vi "LogScaledMessagesOutput.vi"(11 "data out":dbl[](array[numeric])) -> ()   [LabVIEW 2015, in "Diagnostics Addon Engine.lvlib"]
uses:
  Diagnostics Addon Engine.lvlib
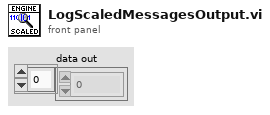
[diagram p1: front panel]
types:
  T1 = enum16{"open", "replace", "create", "open or create", "replace or create", "replace or create with confirmation"}
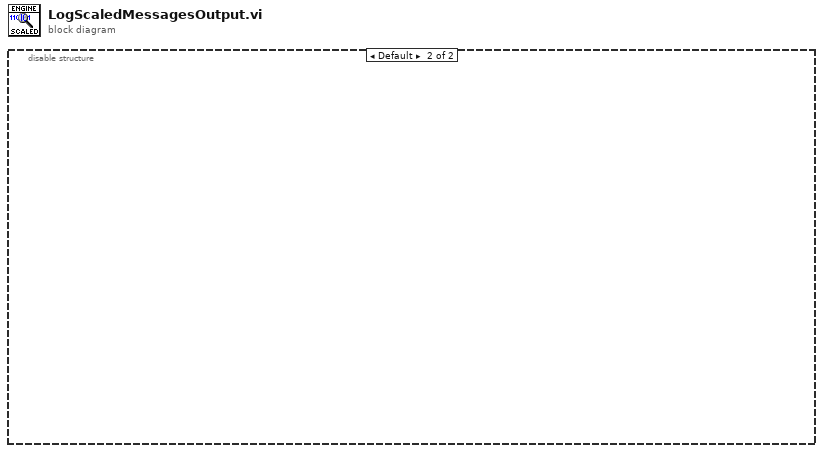
[diagram p0: block diagram]
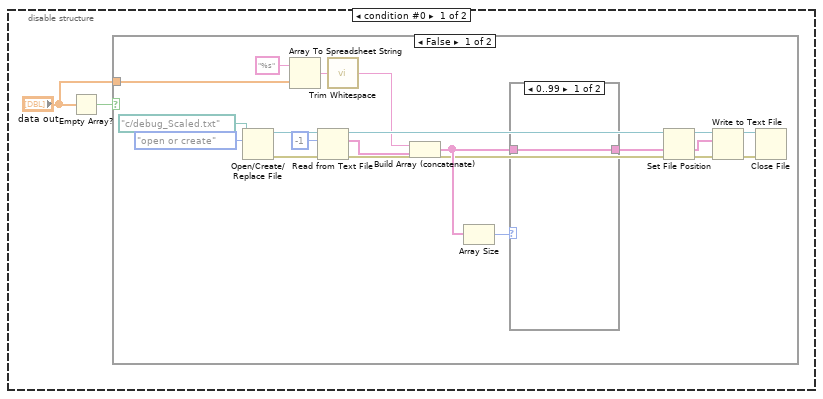
[diagram p2: hidden frame]
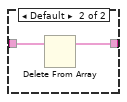
[diagram p3: hidden frame]
diagram:
  n1 = disable-structure shown="Default" {
    frame condition #0 {
      n2 = Empty Array?(array="data out") -> (empty?=w1:bool)
      n3 = case shown="False" w1 {
        tunnel: "data out" -> [w15 _]
        frame False {
          n4 = Open/Create/Replace File(file path (use dialog)=path "c:/debug_Scaled.txt", operation (0:open)=T1."open or create") -> (refnum out=w18:refnum<file>, error out=w19:errorcluster)  [unwired: 4 in, 1 out]
          n5 = Array To Spreadsheet String(array=w15, 3:"%s" ("format string")) -> (spreadsheet string=w13:string)  [unwired: 1 in]
          n6 = Read from Text File(file (use dialog)=w18, count=-1, error in=w19) -> (refnum out=w9:refnum<file>, text=w16:string[], error out=w7:errorcluster)  [unwired: 1 in, 1 out]
          n7 = call <vilib>:"Trim Whitespace.vi"("string"=w13) -> ("trimmed string"=w3:string)  [unwired: 1 in]
          n8 = Build Array (concatenate)(w3, w16) -> (w11:string[])
          n9 = Array Size(array=w11) -> (size(s)=w12:i32)
          n10 = case shown="0..99" w12 {
            tunnel: w11 -> [w22 w24]
            tunnel: [w22 w23] -> w10
            frame 0..99 {
            }
            frame Default {
              n11 = Delete From Array(array=w24) -> (array with subset deleted=w23:string[])  [unwired: 2 in, 1 out]
            }
          }
          n12 = Set File Position(refnum=w9, error in=w7) -> (refnum out=w8:refnum<file>, error out=w6:errorcluster)  [unwired: 2 in]
          n13 = Write to Text File(file (use dialog)=w8, text=w10, error in=w6) -> (refnum out=w4:refnum<file>, error out=w5:errorcluster)  [unwired: 1 in, 1 out]
          n14 = Close File(refnum=w4, error in=w5) -> ()  [unwired: 2 out]
        }
        frame True {
        }
      }
    }
    frame condition #1 (active) {
    }
  }
